vi "GraphLegendGenV2.vi"(4 "Échelle Y":u32[](array[numeric]), 5 "Point":u8[](array[numeric])=[0, 0, 0, 0, 0, 0, 0, 0, 0, 0, 0, 0, 0, 0, 0, 0, 0, 0, 0, 0, 0, 0, 0, 0, 0, 0, 0, 0, 0, 0, 0, 0, 0, 0, 0, 0, 0, 0, 0, 0, 0, 0, 0, 0, 0, 0, 0, 0, 0, 0, 0, 0, 0, 0, 0, 0, 0, 0, 0, 0, 0, 0, 0, 0, 0, 0, 0, 0, 0, 0, 0, 0, 0, 0, 0, 0, 0, 0, 0, 0, 0, 0, 0, 0, 0, 0, 0, 0, 0, 0, 0, 0, 0, 0, 0, 0, 0, 0, 0, 0, 4], 6 "Plot colors":u32[](array[colorbox])=[16777215, 16711680, 65280, 16776960, 65535, 16711935, 255, 16744448, 8388863, 11645283, 46096, 12632256, 34502, 16711808, 9947136, 11826176, 11796589, 7439103, 15728520, 16764921, 61349, 16764296, 12058457, 10539775, 13872565, 16746727, 41215, 8978944, 16757081, 16766208, 10777087, 10066329, 15000804, 13128704, 16760248, 16742466, 13827929, 46140, 10527356, 16777215, 16711680, 65280, 16776960, 65535, 16711935, 255, 16744448, 8388863, 11645283, 46096, 12632256, 34502, 16711808, 9947136, 11826176, 11796589, 7439103, 15728520, 16764921, 61349, 16764296, 12058457, 10539775, 13872565, 16746727, 41215, 8978944, 16757081, 16766208, 10777087, 10066329, 15000804, 13128704, 16760248, 16742466, 13827929, 46140, 10527356, 16777215, 16711680, 65280, 16776960, 65535, 16711935, 255, 16744448, 8388863, 11645283, 46096, 12632256, 34502, 16711808, 9947136, 11826176, 11796589, 7439103, 15728520, 16764921, 61349, 16764296, 12058457, 10539775, 13872565, 16746727, 41215, 8978944, 16757081, 16766208, 10777087, 10066329, 15000804, 13128704, 16760248, 16742466, 13827929, 46140, 10527356, 16777215, 16711680, 65280, 16776960, 65535, 16711935, 255, 16744448, 8388863, 11645283, 46096, 12632256, 34502, 16711808, 9947136, 11826176, 11796589, 7439103, 15728520, 16764921, 61349, 16764296, 12058457, 10539775, 13872565, 16746727, 41215, 8978944, 16757081, 16766208, 10777087, 10066329, 15000804, 13128704, 16760248, 16742466, 13827929, 46140, 10527356], 7 "LastCrvInd":i32=-1, 8 "error in (no error)":errorcluster, 9 "Scan list":string[](array[string]), 10 "Échelle X":string, 11 "XY Graph Ref":refnum<vi>) -> (0 "error out":errorcluster, 1 "Plot colors Out":u32[](array[colorbox])=[16777215, 16711680, 65280, 16776960, 65535, 16711935, 255, 16744448, 8388863, 11645283, 46096, 12632256, 34502, 16711808, 9947136, 11826176, 11796589, 7439103, 15728520, 16764921, 61349, 16764296, 12058457, 10539775, 13872565, 16746727, 41215, 8978944, 16757081, 16766208, 10777087, 10066329, 15000804, 13128704, 16760248, 16742466, 13827929, 46140, 10527356])   [LabVIEW 2010]
doc: "Ce VI formatte la légende du graphique en fonction des paramètres de balayage choisis."
panel:
  in  "Échelle X":u32[](array[numeric])
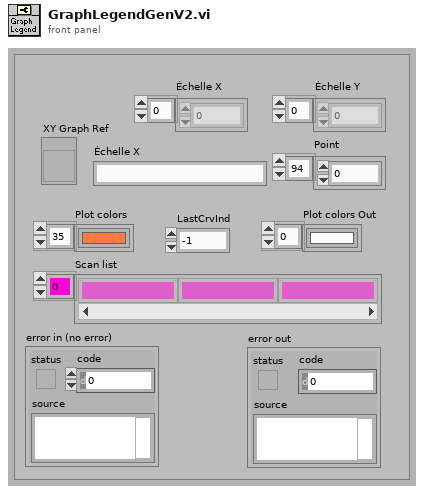
[diagram p1: front panel]
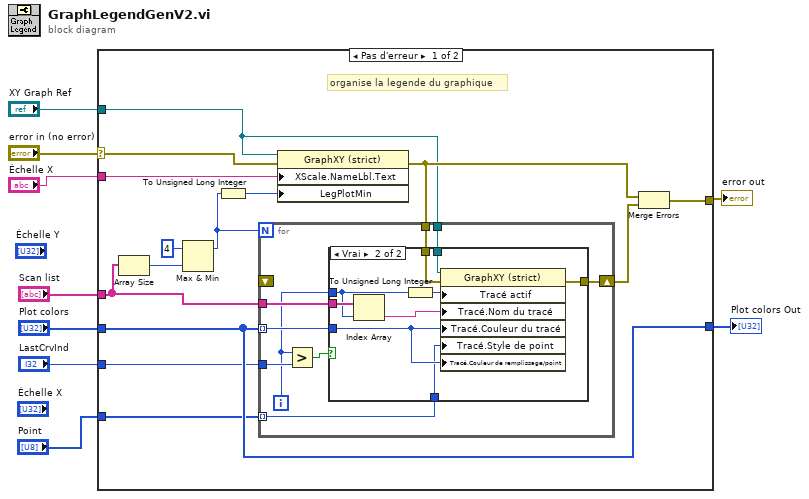
[diagram p0: block diagram]
diagram:
  n1 = case shown="Pas d'erreur" "error in (no error)" {
    selector: "error in (no error)" -> [w12 w44]
    tunnel: "XY Graph Ref" -> [w14 _]
    tunnel: "Scan list" -> [w21 _]
    tunnel: [w22 w44] -> w8
    tunnel: "Plot colors" -> [w15 w43]
    tunnel: [w15 w43] -> w4
    tunnel: "LastCrvInd" -> [w13 _]
    tunnel: "Échelle X" -> [w11 _]
    tunnel: "Point" -> [w10 _]
    frame No Error {
      # "organise la legende du graphique"
      n2 = Array Size(array=w21) -> (size(s)=w20:i32)
      n3 = Max & Min(x=4, y=w20) -> (max(x,y)=w17:i32)  [unwired: 1 out]
      n4 = To Unsigned Long Integer(number=w17) -> (unsigned 32bit integer=w16:u32)
      n5 = property class="GraphXY (strict)"(reference=w14, error in=w12, "XScale.NameLbl.Text"=w11, "LegPlotMin"=w16) -> (error out=w18:errorcluster)  [unwired: 1 out]
      n6 = for {
        N: w17 -> [_]
        tunnel: w21 -> [w28]
        tunnel: w14 -> [w32]
        tunnel: w15 -> [w29] mode=indexing
        tunnel: w18 -> [w31]
        shift-right: [w30] -> w23
        shift-left: _ -> [_]
        tunnel: w13 -> [w27]
        tunnel: w10 -> [w24] mode=indexing
        i -> [w26]
        n7 = Greater?(x=w26, y=w27) -> (0:w25:bool)
        n8 = case shown="Vrai" w25 {
          tunnel: w32 -> [_ w42]
          tunnel: w31 -> [w33 w41]
          tunnel: [w33 w40] -> w30
          tunnel: w29 -> [_ w38]
          tunnel: w26 -> [_ w35]
          tunnel: w28 -> [_ w37]
          tunnel: w24 -> [_ w34]
          frame False {
          }
          frame True {
            n9 = Index Array(array=w37, index=w35) -> (element=w36:string)
            n10 = To Unsigned Long Integer(number=w35) -> (unsigned 32bit integer=w39:u32)
            n11 = property class="GraphXY (strict)"(reference=w42, error in=w41, "Tracé actif"=w39, "Tracé.Nom du tracé"=w36, "Tracé.Couleur du tracé"=w38, "Tracé.Style de point"=w34, "Tracé.Couleur de remplissage/point"=w38) -> (error out=w40:errorcluster)  [unwired: 1 out]
          }
        }
      }
      n12 = Merge Errors(w18, w23) -> (w22:errorcluster)
    }
    frame Error {
    }
  }
  "error out" <- w8
  "Plot colors Out" <- w4
